vi "Teleop.vi"(10 "Match Info":T1={"Autonomous Elapsed Seconds"=0.0, "TeleOp Elapsed Seconds"=0.0, "Disabled Elapsed Seconds"=0.0, "Visited Autonomous"=FALSE, "Visited TeleOp"=FALSE, "Visited Disabled"=FALSE, "Autonomous Settings"={"Autonomous Style"=enum."Independent", "VI Refnum"=refnum}}, 11 "Call Context":T2) -> ()   [LabVIEW 2012]
doc: "This VI is called for each TeleOp packet received from the DS where the robot is not disabled. It is often used to read from the joysticks and update I/O or to update setpoints for timed control loops. It should complete and return within 20 milliseconds or it may miss DS packets."
uses:
  <vilib>/Rock Robotics/WPI/DriverStation/WPI_DriverStationDerivedRobotMode.ctl
  <vilib>/Rock Robotics/WPI/DriverStation/WPI_DriverStationMatch Info.ctl
  Robot Global Data.vi
  <vilib>/Rock Robotics/WPI/Joystick/WPI_JoystickGetSetRefNum.vi
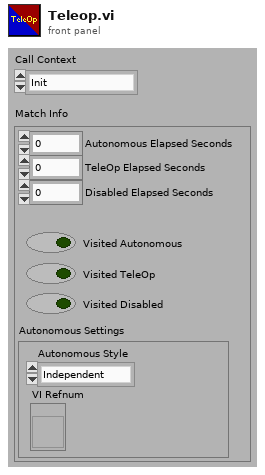
[diagram p1: front panel]
types:
  T1 = typedef "WPI_DriverStationMatch Info.ctl" = cluster{"Autonomous Elapsed Seconds":dbl, "TeleOp Elapsed Seconds":dbl, "Disabled Elapsed Seconds":dbl, "Visited Autonomous":bool, "Visited TeleOp":bool, "Visited Disabled":bool, "Autonomous Settings":cluster{"Autonomous Style":enum16{"Iterative", "Independent"}, "VI Refnum":refnum<vi>}}
  T2 = typedef "WPI_DriverStationDerivedRobotMode.ctl" = enum16{"Init", "Execute", "Stop"}
  T3 = cluster{"JoystickRefnum":string, "Axis":u8, "Deadband":dbl}
  T4 = typedef "WPI_JoystickDevRef.ctl" = cluster{"Device":T5}
  T5 = typedef "WPI_JoystickDeviceEnum.ctl" = enum16{"USB 1", "USB 2", "USB 3", "USB 4", "Kinect 1", "Kinect 2"}
  T6 = typedef "WPI_JoystickButtonState.ctl" = cluster{"Button 1":bool, "Button 2":bool, "Button 3":bool, "Button 4":bool, "Button 5":bool, "Button 6":bool, "Button 7":bool, "Button 8":bool, "Button 9":bool, "Button 10":bool, "Button 11":bool, "Button 12":bool}
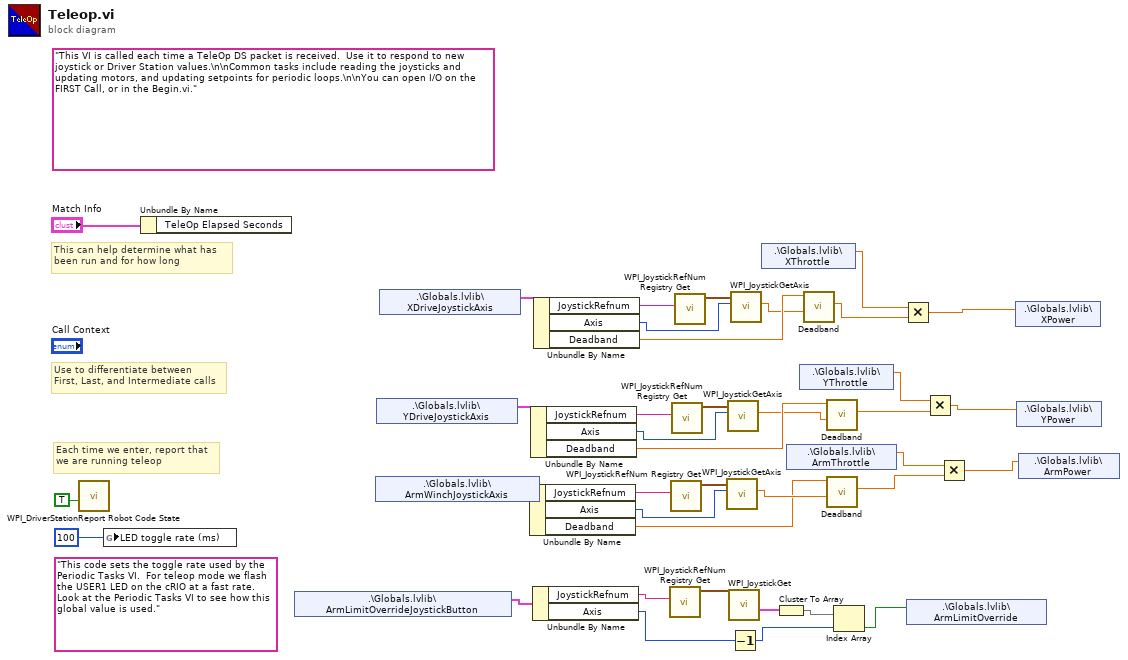
[diagram p0: block diagram]
diagram:
  (unwired) "This code sets the toggle rate used by the Periodic Tasks VI.  For teleop mode we flash the USER1 LED on the cRIO at a fast rate.  Look at the Periodic Tasks VI to see how this global value is used."
  (unwired) "This VI is called each time a TeleOp DS packet is received.  Use it to respond to new joystick or Driver Station values.\n\nCommon tasks include reading the joysticks and updating motors, and updating setpoints for periodic loops.\n\nYou can open I/O on the FIRST Call, or in the Begin.vi."
  # "Each time we enter, report that\nwe are running teleop"
  # "Use to differentiate between\nFirst, Last, and Intermediate calls"
  # "This can help determine what has\nbeen run and for how long"
  n1 = call <vilib>:"WPI_DriverStationReport Robot Code State.vi"("TeleOp"=TRUE ("Autonomous")) -> ()  [unwired: 10 in, 1 out]
  n2 = global write "Robot Global Data.vi" "LED toggle rate (ms)"(u32 100 ("LED ms toggle rate")) -> ()
  n3 = Unbundle By Name("Match Info") -> ()  [unwired: 1 out]
  n4 = shared-variable ".\\Globals.lvlib\\ArmLimitOverrideJoystickButton"() -> (w8:cluster{"JoystickRefnum":string, "Axis":u8})  [unwired: 1 in, 1 out]
  n5 = shared-variable ".\\Globals.lvlib\\ArmWinchJoystickAxis"() -> (w21:T3)  [unwired: 1 in, 1 out]
  n6 = shared-variable ".\\Globals.lvlib\\YDriveJoystickAxis"() -> (w22:T3)  [unwired: 1 in, 1 out]
  n7 = shared-variable ".\\Globals.lvlib\\XDriveJoystickAxis"() -> (w29:T3)  [unwired: 1 in, 1 out]
  n8 = Unbundle By Name(w21) -> ("JoystickRefnum"=w20:string, "Axis"=w18:u8, "Deadband"=w14:dbl)
  n9 = Unbundle By Name(w22) -> ("JoystickRefnum"=w23:string, "Axis"=w25:u8, "Deadband"=w17:dbl)
  n10 = Unbundle By Name(w8) -> ("JoystickRefnum"=w7:string, "Axis"=w4:u8)
  n11 = Unbundle By Name(w29) -> ("JoystickRefnum"=w28:string, "Axis"=w26:u8, "Deadband"=w10:dbl)
  n12 = call <vilib>:"WPI_JoystickRefNum Registry Get.vi"("refnum name"=w7) -> ("JoystickDevRef"=w6:T4)  [unwired: 9 in, 1 out]
  n13 = call <vilib>:"WPI_JoystickRefNum Registry Get.vi"("refnum name"=w20) -> ("JoystickDevRef"=w19:T4)  [unwired: 9 in, 1 out]
  n14 = call <vilib>:"WPI_JoystickRefNum Registry Get.vi"("refnum name"=w23) -> ("JoystickDevRef"=w24:T4)  [unwired: 9 in, 1 out]
  n15 = call <vilib>:"WPI_JoystickRefNum Registry Get.vi"("refnum name"=w28) -> ("JoystickDevRef"=w27:T4)  [unwired: 9 in, 1 out]
  n16 = call <vilib>:"WPI_JoystickGetAxis.vi"("Axis"=w18, "JoystickDevRef"=w19) -> ("Value"=w15:dbl)  [unwired: 8 in, 1 out]
  n17 = call <vilib>:"WPI_JoystickGetAxis.vi"("Axis"=w25, "JoystickDevRef"=w24) -> ("Value"=w16:dbl)  [unwired: 8 in, 1 out]
  n18 = call <vilib>:"WPI_JoystickGet.vi"("JoystickDevRef"=w6) -> ("Buttons"=w5:T6)  [unwired: 4 in, 2 out]
  n19 = Decrement(x=w4) -> (x-1=w2:u8)
  n20 = call <vilib>:"WPI_JoystickGetAxis.vi"("Axis"=w26, "JoystickDevRef"=w27) -> ("Value"=w9:dbl)  [unwired: 8 in, 1 out]
  n21 = shared-variable ".\\Globals.lvlib\\XThrottle"() -> (w35:dbl)  [unwired: 1 in, 1 out]
  n22 = Cluster To Array(cluster=w5) -> (array=w3:bool[])
  n23 = shared-variable ".\\Globals.lvlib\\ArmThrottle"() -> (w31:dbl)  [unwired: 1 in, 1 out]
  n24 = shared-variable ".\\Globals.lvlib\\YThrottle"() -> (w33:dbl)  [unwired: 1 in, 1 out]
  n25 = call "Deadband.vi"("Input"=w9, "Deadband"=w10) -> ("Output"=w11:dbl)  [unwired: 9 in]
  n26 = call "Deadband.vi"("Input"=w16, "Deadband"=w17) -> ("Output"=w12:dbl)  [unwired: 9 in]
  n27 = call "Deadband.vi"("Input"=w15, "Deadband"=w14) -> ("Output"=w13:dbl)  [unwired: 9 in]
  n28 = Index Array(array=w3, index=w2) -> (element=w1:bool)
  n29 = Multiply(x=w35, y=w11) -> (x*y=w34:dbl)
  n30 = shared-variable ".\\Globals.lvlib\\ArmLimitOverride"(w1) -> ()  [unwired: 1 in, 1 out]
  n31 = Multiply(x=w33, y=w12) -> (x*y=w32:dbl)
  n32 = Multiply(x=w31, y=w13) -> (x*y=w30:dbl)
  n33 = shared-variable ".\\Globals.lvlib\\XPower"(w34) -> ()  [unwired: 1 in, 1 out]
  n34 = shared-variable ".\\Globals.lvlib\\YPower"(w32) -> ()  [unwired: 1 in, 1 out]
  n35 = shared-variable ".\\Globals.lvlib\\ArmPower"(w30) -> ()  [unwired: 1 in, 1 out]
